vi "XML Edit.vi"(5 "New Value":u32, 6 "error in (no error)":errorcluster, 7 "Data Type":string, 8 "Parameter":string, 9 "XML in":string) -> (0 "error out":errorcluster, 3 "XML out":string)   [LabVIEW 2021, in "BS120x Driver.lvlib" / "ENET_BS1200.lvclass"]
uses:
  ENET_BS1200.lvclass
  <vilib>/xml/Close Reference(Node).vi
  <resource>/objmgr/DOMUserDefRef.rc
  <vilib>/xml/NI_XML.lvlib
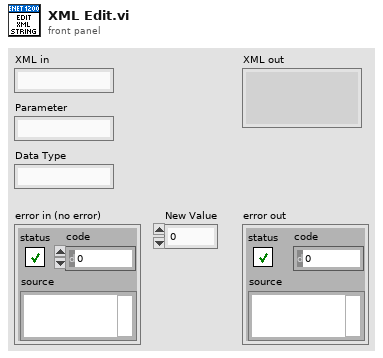
[diagram p1: front panel]
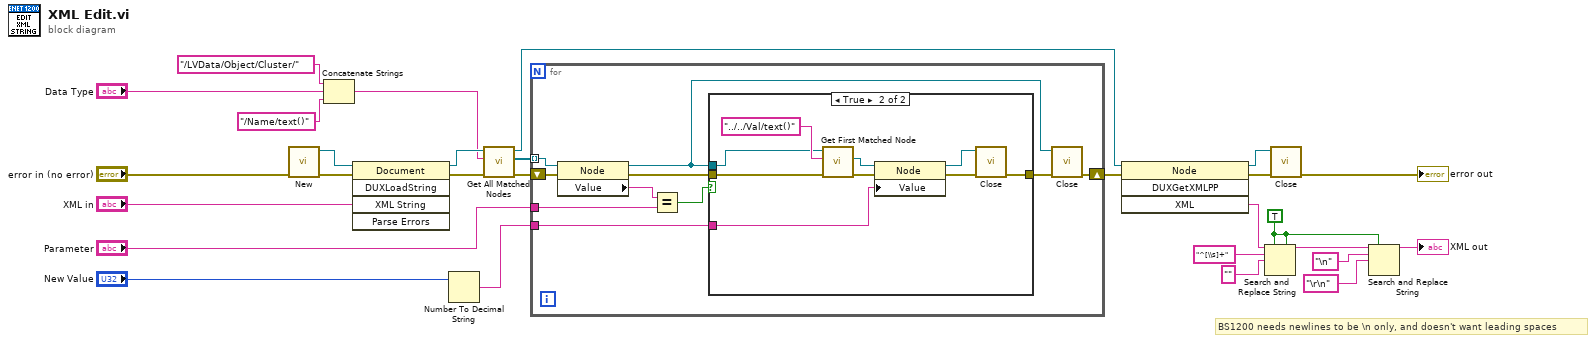
[diagram p0: block diagram]
diagram:
  w5 = TRUE ("replace all? (F)")
  # "BS1200 needs newlines to be \\n only, and doesn't want leading spaces"
  n1 = call <vilib>:"New.vi"("error in (no error)"="error in (no error)") -> ("error out"=w27:errorcluster, "DOM document out"=w28:refnum<k20>)  [unwired: 7 in]
  n2 = Concatenate Strings("/LVData/Object/Cluster/" ("XPath expression"), "Data Type", "/Name/text()" ("string")) -> (w16:string)
  n3 = invoke class="Document" method="DUXLoadString"(reference=w28, error in=w27, "XML String"="XML in") -> (reference out=w24:refnum<k20>, error out=w25:errorcluster)  [unwired: 2 in, 3 out]
  n4 = Number To Decimal String(number="New Value") -> (decimal integer string=w17:string)  [unwired: 1 in]
  n5 = call <vilib>:"Get All Matched Nodes.vi"("error in (no error)"=w25, "XPath expression"=w16, "node in"=w24) -> ("error out"=w23:errorcluster, "node result array"=w22:refnum<k20>[], "node out"=w1:refnum<k20>)  [unwired: 6 in]
  n6 = for {
    shift-right: [w33] -> w21
    shift-left: w23 -> [w38]
    tunnel: w22 -> [w37] mode=indexing
    tunnel: w17 -> [w32]
    tunnel: "Parameter" -> [w31]
    n7 = property class="Node"(reference=w37, error in=w38) -> (reference out=w35:refnum<k20>, error out=w36:errorcluster, "Value"=w30:string)
    n8 = Equal?(x=w30, y=w31) -> (x = y?=w29:bool)
    n9 = case shown="True" w29 {
      tunnel: w35 -> [_ w42]
      tunnel: w36 -> [w39 w46]
      tunnel: [w39 w41] -> w34
      tunnel: w32 -> [_ w40]
      frame False {
      }
      frame True {
        n10 = call <vilib>:"Get First Matched Node.vi"("error in (no error)"=w46, "XPath expression"="../../Val/text()", "node in"=w42) -> ("error out"=w44:errorcluster, "node result"=w43:refnum<k20>)  [unwired: 6 in, 1 out]
        n11 = property class="Node"(reference=w43, error in=w44, "Value"=w40) -> (reference out=w47:refnum<k20>, error out=w48:errorcluster)
        n12 = call-poly <vilib>:"Close.vi"("error in (no error)"=w48, "node"=w47) -> ("error out"=w41:errorcluster)  [unwired: 7 in]
      }
    }
    n13 = call-poly <vilib>:"Close.vi"("error in (no error)"=w34, "node"=w35) -> ("error out"=w33:errorcluster)  [unwired: 7 in]
  }
  n14 = invoke class="Node" method="DUXGetXMLPP"(reference=w1, error in=w21) -> (reference out=w19:refnum<k20>, error out=w20:errorcluster, "XML"=w9:string)  [unwired: 2 in, 1 out]
  n15 = Search and Replace String(replace all?=w5, multiline?=w5, input string=w9, search string="^[\\s]+", replace string="" ("search string")) -> (result string=w6:string)  [unwired: 3 in, 3 out]
  n16 = call-poly <vilib>:"Close.vi"("error in (no error)"=w20, "node"=w19) -> ("error out"=→"error out":errorcluster)  [unwired: 7 in]
  n17 = Search and Replace String(replace all?=w5, input string=w6, search string="\n", replace string="\r\n" ("search string")) -> (result string=→"XML out":string)  [unwired: 4 in, 3 out]
